vi "Apply SDI to Word.vi"(7 "sdi":u8, 11 "word in":u32) -> (3 "word out":u32)   [LabVIEW 2020, in "Ballard ARINC 429 Engine.lvlib" / "Implementation.lvlib" / "Tx Acyclic Labels Execution Unit.lvclass"]
uses:
  Tx Acyclic Labels Execution Unit.lvclass
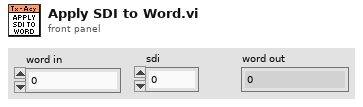
[diagram p1: front panel]
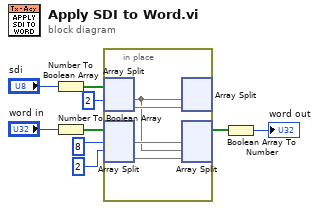
[diagram p0: block diagram]
diagram:
  n1 = Number To Boolean Array(number="sdi") -> (Boolean array=w2:bool[])
  n2 = Number To Boolean Array(number="word in") -> (Boolean array=w7:bool[])
  n3 = in-place {
    n4 = in-place-split #1(w2, 2) -> (w10:bool[], w11:bool[])
    n5 = in-place-split #2(w7, 8, 2) -> (w13:bool[], w12:bool[])  [unwired: 1 out]
    n6 = in-place-split #1(w10, w11) -> ()  [unwired: 2 out]
    n7 = in-place-split #2(w13, w10, w12) -> (w6:bool[])  [unwired: 2 out]
  }
  n8 = Boolean Array To Number(Boolean array=w6) -> (number=→"word out":u32)
